vi "Drive Straight.vi"(3 "reinitialize? (F)":bool, 4 "Maneuver":T2(ring), 5 "Turn Setpoint":dbl, 7 "PID gains M":T1, 8 "Drive Setpoint":dbl, 9 "Angle":dbl, 10 "Angle to Get":dbl, 11 "Enable?":bool) -> (1 "Turn Setpoint":dbl)   [LabVIEW 2019]
uses:
  <vilib>/addons/control/pid/pid.llb/PID (DBL).vi
  <vilib>/addons/control/pid/NI_PID_pid.lvlib
panel:
  out "Waveform Chart":cluster{dbl, dbl}(graph)
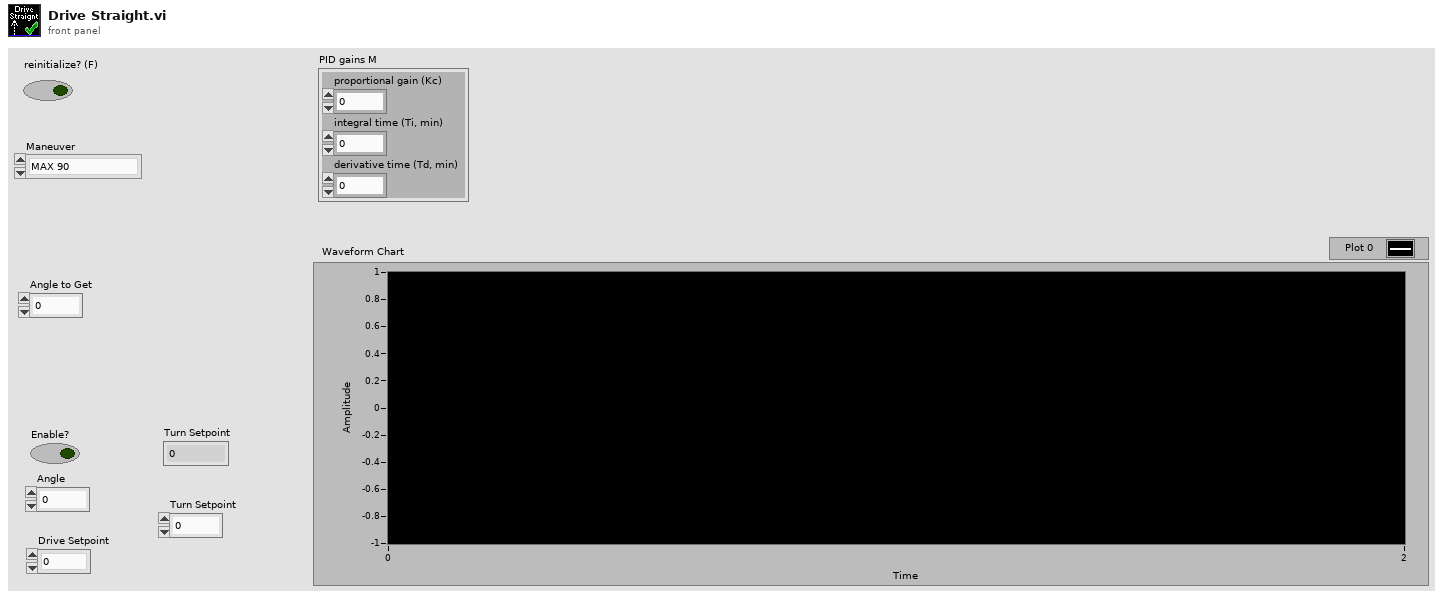
[diagram p1: front panel]
types:
  T1 = cluster{"proportional gain (Kc)":dbl, "integral time (Ti, min)":dbl, "derivative time (Td, min)":dbl}
  T2 = enum16{"MAX 90", "Pod Racer", "MAX 180", "Turn to Home", "Turn to Rocket", "Auto-Align", "Turn to ..."}
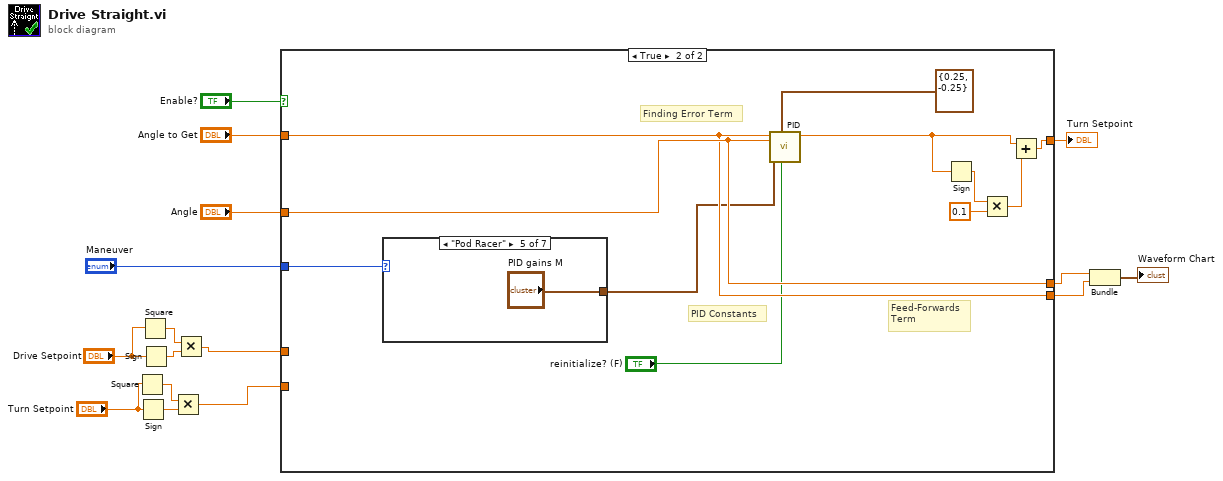
[diagram p0: block diagram]
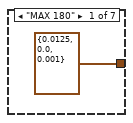
[diagram p3: hidden frame]
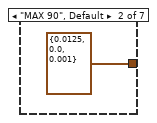
[diagram p4: hidden frame]
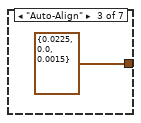
[diagram p5: hidden frame]
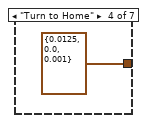
[diagram p6: hidden frame]
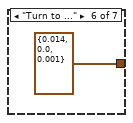
[diagram p7: hidden frame]
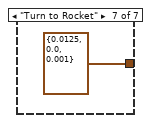
[diagram p8: hidden frame]
diagram:
  n1 = Square(x="Turn Setpoint") -> (x^2=w12:dbl)
  n2 = Sign(1:"Turn Setpoint") -> (0:w11:dbl)
  n3 = Square(x="Drive Setpoint") -> (x^2=w9:dbl)
  n4 = Sign(1:"Drive Setpoint") -> (0:w8:dbl)
  n5 = Multiply(x=w12, y=w11) -> (x*y=w10:dbl)
  n6 = Multiply(x=w9, y=w8) -> (x*y=w7:dbl)
  n7 = case shown="True" "Enable?" {
    tunnel: [w17 w20] -> w2
    tunnel: "Angle" -> [_ w27]
    tunnel: w7 -> [_ _]
    tunnel: "Angle to Get" -> [_ w26]
    tunnel: w10 -> [w17 _]
    tunnel: [_ w27] -> w4
    tunnel: [_ w26] -> w3
    tunnel: "Maneuver" -> [_ w24]
    frame False {
    }
    frame True {
      # "Feed-Forwards\nTerm"
      # "PID Constants"
      # "Finding Error Term"
      n8 = case shown="\"Pod Racer\"" w24 {
        tunnel: [T1 {"proportional gain (Kc)"=0.0125, "integral time (Ti, min)"=0.0, "derivative time (Td, min)"=0.001} ("PID gains M") T1 {"proportional gain (Kc)"=0.0125, "integral time (Ti, min)"=0.0, "derivative time (Td, min)"=0.001} ("PID gains M") T1 {"proportional gain (Kc)"=0.0225, "integral time (Ti, min)"=0.0, "derivative time (Td, min)"=0.0015} ("PID gains M") T1 {"proportional gain (Kc)"=0.0125, "integral time (Ti, min)"=0.0, "derivative time (Td, min)"=0.001} ("PID gains M") "PID gains M" T1 {"proportional gain (Kc)"=0.014, "integral time (Ti, min)"=0.0, "derivative time (Td, min)"=0.001} ("PID gains M") T1 {"proportional gain (Kc)"=0.0125, "integral time (Ti, min)"=0.0, "derivative time (Td, min)"=0.001} ("PID gains M")] -> w23
        frame "MAX 180" {
        }
        frame "MAX 90", Default {
        }
        frame "Auto-Align" {
        }
        frame "Turn to Home" {
        }
        frame "Pod Racer" {
        }
        frame "Turn to ..." {
        }
        frame "Turn to Rocket" {
        }
      }
      n9 = call-poly <vilib>:"PID.vi"("reinitialize? (F)"="reinitialize? (F)", "output range"=cluster{"output high":dbl, "output low":dbl} {"output high"=0.25, "output low"=-0.25}, "PID gains"=w23, "process variable"=w27, "setpoint"=w26) -> ("output"=w18:dbl)  [unwired: 5 in, 1 out]
      n10 = Sign(1:w18) -> (0:w22:dbl)
      n11 = Multiply(x=w22, y=0.1) -> (x*y=w21:dbl)
      n12 = Add(x=w18, y=w21) -> (x+y=w20:dbl)
    }
  }
  "Turn Setpoint" <- w2
  n13 = Bundle("Angle"=w4, "Angle to Get"=w3) -> (→"Waveform Chart":cluster{"Angle":dbl, "Angle to Get":dbl})  [unwired: 1 in]
